vi "Begin.vi"(8 "error in":errorcluster) -> (0 "error out":errorcluster)   [LabVIEW 2014]
doc: "Called before other user functions, this VI is expected to open initial I/O refnums, load in file data, and do all program initialization. Notice that the <B>error out</B> terminal is simply used for data flow. Wiring it to other structures or subVIs ensures that this VI runs first."
uses:
  <vilib>/Rock Robotics/SystemInterfaces/DIO/FPGA_DIOPWMChannel.ctl
  <vilib>/Rock Robotics/WPI/SafetyOutput/WPI_SafetyOutputConfigMenu.ctl
  <vilib>/Rock Robotics/WPI/DriverStation/WPI_DriverStationRobotMode2.ctl
  <vilib>/Rock Robotics/WPI/Joystick/WPI_JoystickDeviceEnum.ctl
  <vilib>/Rock Robotics/WPI/Encoder/WPI_EncoderType.ctl
  <vilib>/Rock Robotics/WPI/RobotDrive/WPI_RobotDriveOpen2MotorWithTalon.vi
  Robot Global Data.vi
  <vilib>/Rock Robotics/Network Tables/SD Write String Array.vi
  <vilib>/Rock Robotics/WPI/MotorControl/WPI_MotorControlOpen Talon.vi
  <vilib>/Rock Robotics/WPI/Solenoid/WPI_SolenoidOpenSingle.vi
  <vilib>/Rock Robotics/WPI/Counter/WPI_CounterDigitalInputToDigitalSource.vi
  LIDAR Present Variable.vi
  <vilib>/express/express arith-compare/Formula/XNode/ExpressFormulaBlockNode.xnode
panel:
  out "Encoder  Ratio 3":dbl
  out "Encoder  Ratio 2":dbl
  out "Encoder  Ratio":dbl
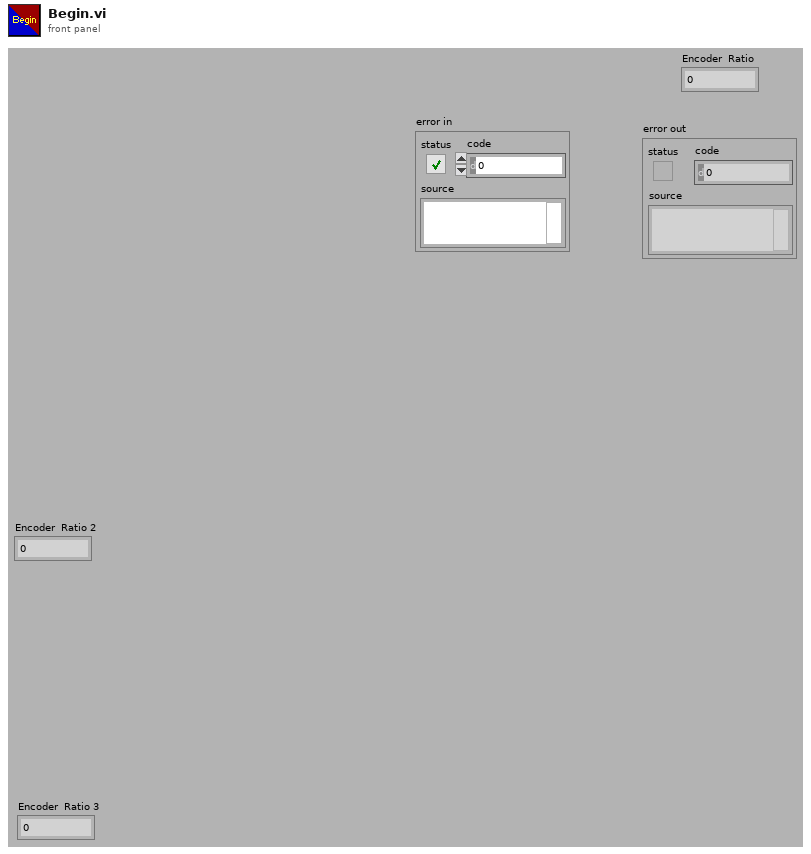
[diagram p1: front panel]
types:
  T1 = enum16{"Solenoid 0", "Solenoid 1", "Solenoid 2", "Solenoid 3", "Solenoid 4"}
  T2 = typedef "WPI_EncoderType.ctl" = enum16{"1x", "2x", "4x"}
  T3 = enum16{"DIO 0", "DIO 1", "DIO 2", "DIO 3", "DIO 4", "DIO 5", "DIO 6", "DIO 7", "DIO 8", "DIO 9"}
  T4 = enum16{"DIO 0", "DIO 1", "DIO 2", "DIO 3", "DIO 4", "DIO 5", "DIO 6", "DIO 7"}
  T5 = enum16{"DIO 0", "DIO 1", "DIO 2", "DIO 3", "DIO 4", "DIO 5", "DIO 6"}
  T6 = typedef "WPI_JoystickDeviceEnum.ctl" = enum16{"USB 0", "USB 1", "USB 2", "USB 3", "USB 4", "USB 5"}
  T7 = enum16{"Solenoid 0", "Solenoid 1", "Solenoid 2", "Solenoid 3", "Solenoid 4", "Solenoid 5"}
  T8 = typedef "FPGA_DIOPWMChannel.ctl" = enum8{"PWM 0", "PWM 1", "PWM 2", "PWM 3", "PWM 4", "PWM 5", "PWM 6", "PWM 7", "PWM 8", "PWM 9", "PWM MXP 0", "PWM MXP 1", "PWM MXP 2", "PWM MXP 3", "PWM MXP 4", "PWM MXP 5", "PWM MXP 6", "PWM MXP 7", "PWM MXP 8", "PWM MXP 9", "Invalid"}
  T9 = typedef "WPI_DriverStationRobotMode2.ctl" = enum16{"Autonomous Disabled", "Autonomous Enabled", "Teleop Disabled", "Teleop Enabled", "Disconnected", "Finish", "Test Disabled", "Test Enabled", "Emergency Stopped"}
  T10 = typedef "WPI_SafetyOutputConfigMenu.ctl" = enum16{"Enable", "Disable"}
  T11 = typedef "WPI_JoystickDevRef.ctl" = cluster{"Device":T6}
  T12 = typedef "WPI_GyroDevRef.ctl" = cluster{"DevStatus":errorcluster, "Analog Module":T13, "Analog Channel":T14, "Offset":dbl, "Gain (VoltsPerDegree/Second)":dbl}
  T13 = typedef "FPGA_TypedefAnalogModule.ctl" = enum16{"Controller 1"}
  T14 = typedef "FPGA_AIChannel.ctl" = enum8{"AI 0", "AI 1", "AI 2", "AI 3", "AI MXP 0", "AI MXP 1", "AI MXP 2", "AI MXP 3", "Invalid"}
  T15 = typedef "WPI_MotorControlDeviceRef.ctl" = cluster{"DeviceStatus":errorcluster, "Type":T16, "PWM":cluster{"Controller":T17, "PWM Channel":T8, "DeadBand":T18}, "CAN":cluster{"Device Number":u8, "Control Mode":T19, "Semaphore":T20, "Max Vout":dbl, "TalonSRX Control Mode":T21}, "Invert":bool, "TransformRef":T22, "InvTransformRef":T22}
  T16 = typedef "WPI_MotorControlType.ctl" = enum16{"PWM", "CAN", "CANTalonSRX"}
  T17 = typedef "FPGA_TypedefDigitalModule.ctl" = enum16{"Controller 1"}
  T18 = typedef "WPI_PWMDeadband.ctl" = cluster{"Name":string, "maxPositivePwm":i32, "minPositivePwm":i32, "centerPwm":i32, "maxNegativePwm":i32, "minNegativePwm":i32, "angularRange":u16}
  T19 = typedef "WPI_CANJaguar_ControlMode.ctl" = enum8{"Percent VBus", "Current", "Speed", "Position", "Voltage"}
  T20 = typedef "Semaphore RefNum" = refnum<k1>
  T21 = typedef "WPI_CANTalonSRX_APIControlMode.ctl" = enum8{"Percent VBus", "Speed", "Position", "Slave", "Unchanged / Invalid"}
  T22 = typedef "WPI_PWMTransform_ConPane.ctl" = refnum<vi>
  T23 = typedef "WPI_RobotDriveDevRef.ctl" = cluster{"DevStatus":errorcluster, "Motors[]":T15[], "Square Inputs":bool, "Max Output":dbl}
  T24 = typedef "WPI_DigitalInputDevRef.ctl" = cluster{"DevStatus":errorcluster, "DIO Channel":T25, "Controller":T17}
  T25 = typedef "FPGA_DIOChannel.ctl" = enum8{"DIO 0", "DIO 1", "DIO 2", "DIO 3", "DIO 4", "DIO 5", "DIO 6", "DIO 7", "DIO 8", "DIO 9", "DIO MXP 0", "DIO MXP 1", "DIO MXP 2", "DIO MXP 3", "DIO MXP 4", "DIO MXP 5", "DIO MXP 6", "DIO MXP 7", "DIO MXP 8", "DIO MXP 9", "DIO MXP 10", "DIO MXP 11", "DIO MXP 12", "DIO MXP 13", "DIO MXP 14", "DIO MXP 15", "Invalid"}
  T26 = typedef "WPI_SolenoidDevRef.ctl" = cluster{"DevStatus":errorcluster, "Pneumatics Control Module":u8, "Forward Solenoid Channel":T27, "Reverse Solenoid Channel":T27}
  T27 = typedef "WPI_SolenoidChannel.ctl" = enum8{"Solenoid 0", "Solenoid 1", "Solenoid 2", "Solenoid 3", "Solenoid 4", "Solenoid 5", "Solenoid 6", "Solenoid 7", "Invalid"}
  T28 = typedef "FPGA_CounterEncoderSourceConvertionLVSourceType.ctl" = cluster{"DevStatus":errorcluster, "AnalogTriggerMode?":bool, "DigitalMode":cluster{"Controller":T17, "DIO Channel":T29}, "AnalogTriggerMode":cluster{"AnalogTriggerIndex":T30, "OutputType":T31}}
  T29 = typedef "FPGA_DIODigitalSourceChannel.ctl" = enum8{"DIO 0", "DIO 1", "DIO 2", "DIO 3", "DIO 4", "DIO 5", "DIO 6", "DIO 7", "DIO 8", "DIO 9", "DIO MXP 0", "DIO MXP 1", "DIO MXP 2", "DIO MXP 3", "DIO MXP 4", "DIO MXP 5", "DIO MXP 6", "DIO MXP 7", "DIO MXP 8", "DIO MXP 9", "DIO MXP 10", "DIO MXP 11", "DIO MXP 12", "DIO MXP 13", "DIO MXP 14", "DIO MXP 15", "Disabled"}
  T30 = typedef "FPGA_AnalogTriggerIndex.ctl" = enum8{"Trig 0", "Trig 1", "Trig 2", "Trig 3", "Trig 4", "Trig 5", "Trig 6", "Trig 7", "Invalid"}
  T31 = typedef "FPGA_AnalogTriggerOutType.ctl" = enum16{"InWindow", "TriggerState", "Rising", "Falling"}
  T32 = typedef "WPI_EncoderDevRef.ctl" = cluster{"DevStatus":errorcluster, "EncoderIndex":T33, "CounterIndex":T34, "DistancePerCount":dbl, "Decoding Type":T2}
  T33 = typedef "FPGA_EncoderIdx.ctl" = enum8{"Enc 0", "Enc 1", "Enc 2", "Enc 3", "Enc 4", "Enc 5", "Enc 6", "Enc 7", "Invalid"}
  T34 = typedef "FPGA_CounterCtrSystemIndex.ctl" = enum8{"Ctr 0", "Ctr 1", "Ctr 2", "Ctr 3", "Ctr 4", "Ctr 5", "Ctr 6", "Ctr 7", "Invalid"}
  T35 = typedef "WPI_I2CDevRef.ctl" = cluster{"DevStatus":errorcluster, "Controller":T17, "Device Address":u8, "Handle":i32, "I2C Bus":T36}
  T36 = typedef "i2c_bus.ctl" = enum16{"I2C On-Board", "I2C MXP", "Invalid"}
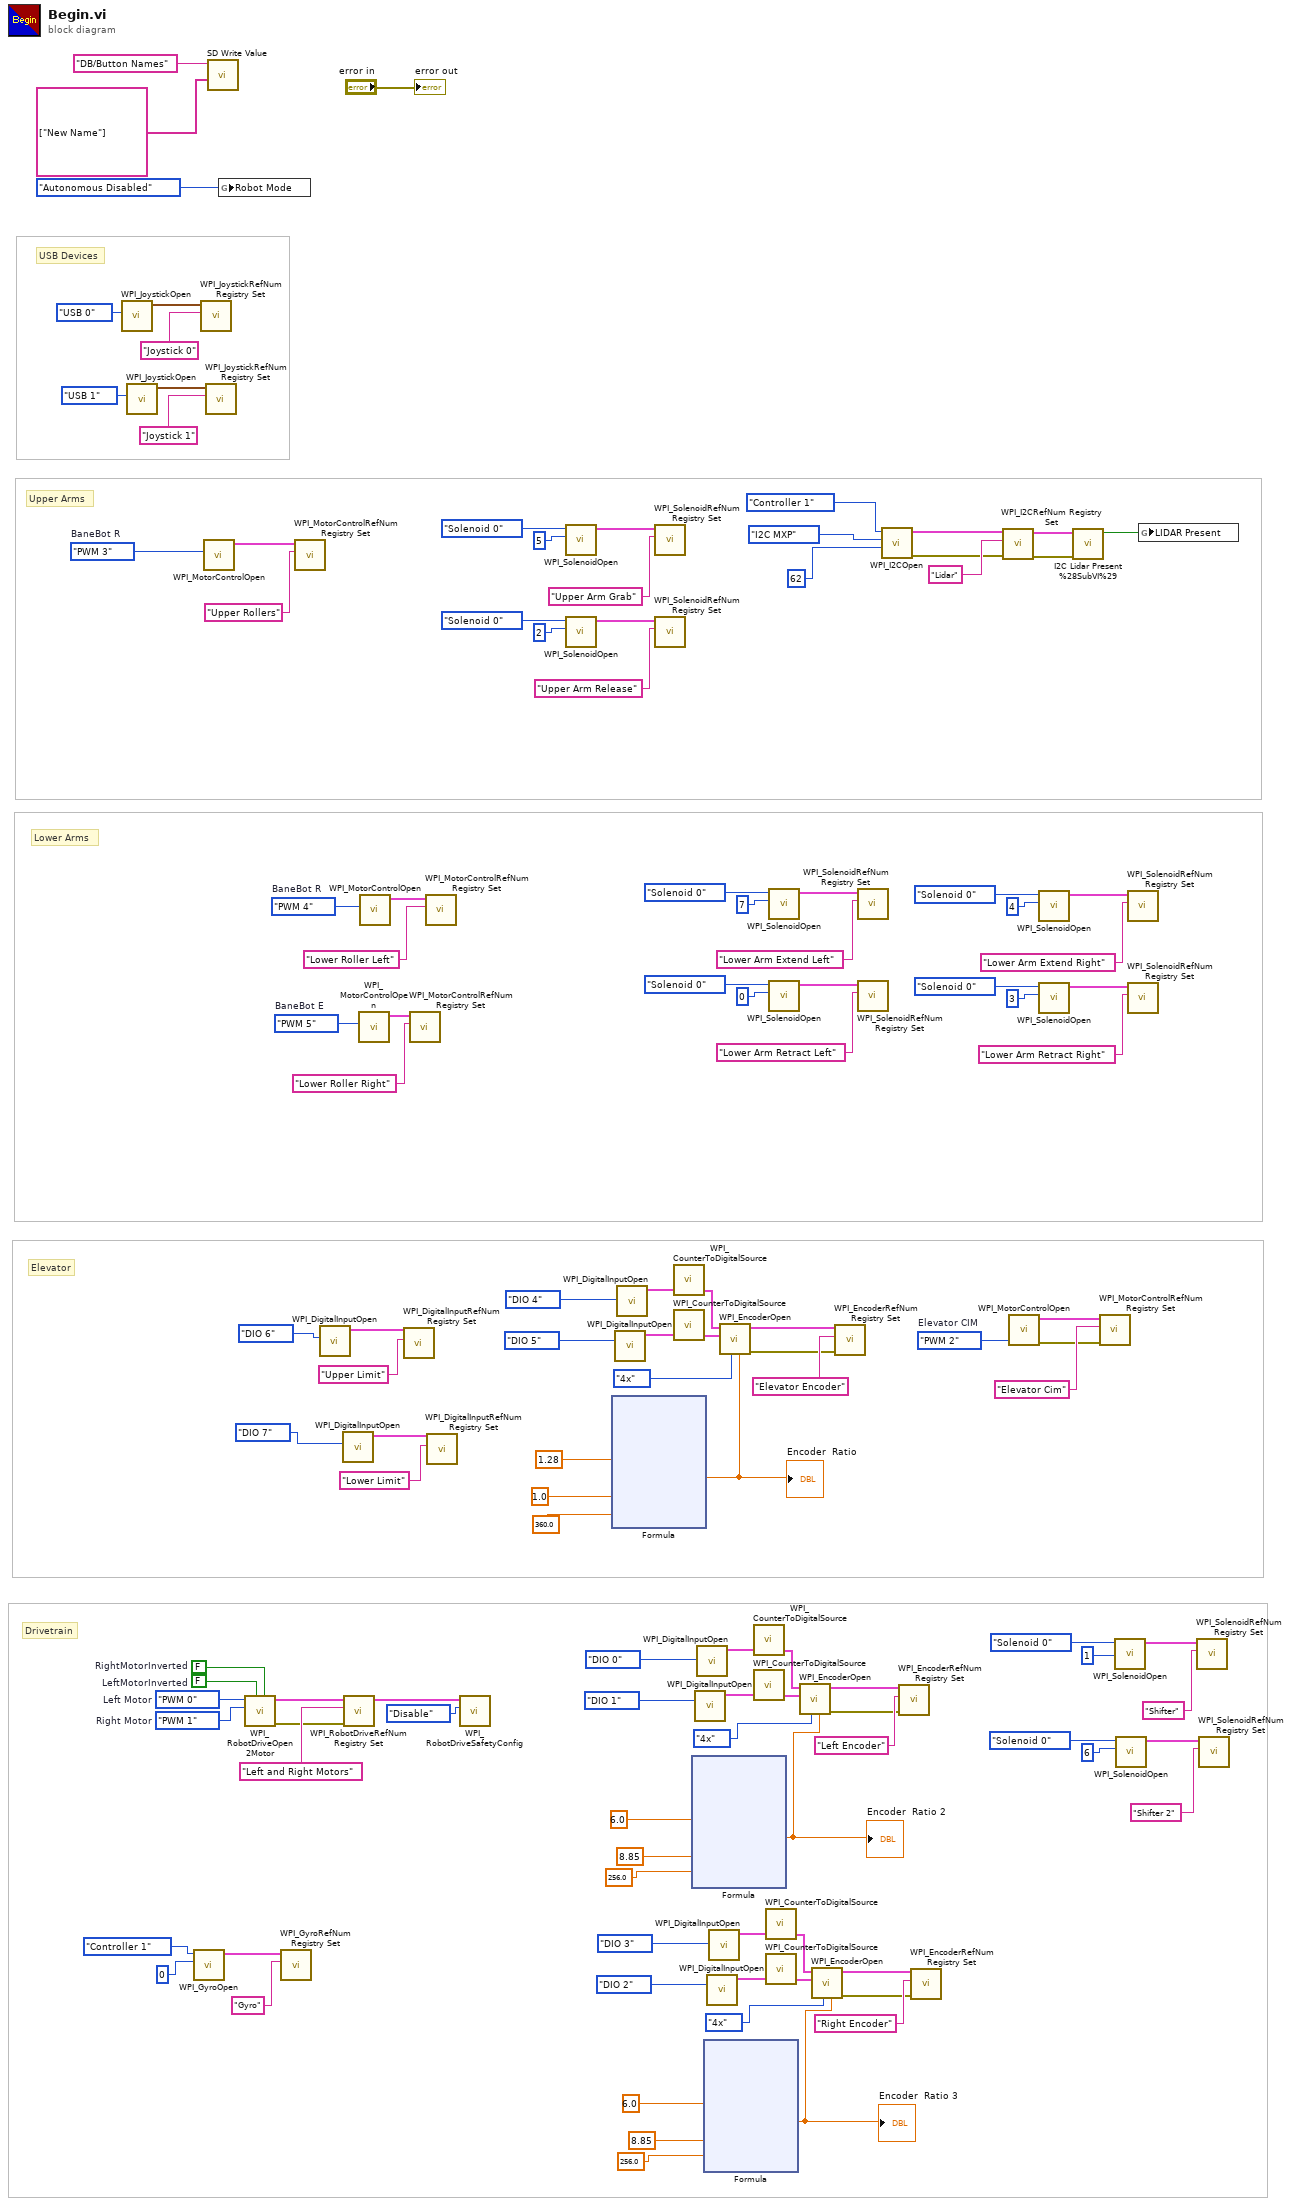
[diagram p0: block diagram]
diagram:
  w98 = FPGA_DIOPWMChannel."PWM 2"  # Elevator CIM
  w102 = FPGA_DIOPWMChannel."PWM 5"  # BaneBot E
  w106 = FPGA_DIOPWMChannel."PWM 4"  # BaneBot R
  w108 = FPGA_DIOPWMChannel."PWM 3"  # BaneBot R
  w119 = FPGA_DIOPWMChannel."PWM 1"  # Right Motor
  w120 = FPGA_DIOPWMChannel."PWM 0"  # Left Motor
  w124 = FALSE  # LeftMotorInverted
  w125 = FALSE  # RightMotorInverted
  # "Upper Arms"
  # "Lower Arms"
  # "Elevator"
  # "Drivetrain"
  # "USB Devices"
  n1 = call <vilib>:"WPI_JoystickOpen.vi"("JoystickDevice"=WPI_JoystickDeviceEnum."USB 0") -> ("JoystickDevRef"=w114:T11)  [unwired: 10 in]
  n2 = call <vilib>:"WPI_JoystickOpen.vi"("JoystickDevice"=WPI_JoystickDeviceEnum."USB 1") -> ("JoystickDevRef"=w79:T11)  [unwired: 10 in]
  n3 = call <vilib>:"WPI_GyroOpen.vi"("Analog Channel"=0, "Controller"=enum16{"Controller 1"}."Controller 1") -> ("GyroDevRef"=w21:T12)  [unwired: 7 in, 2 out]
  n4 = call <vilib>:"WPI_JoystickRefNum Registry Set.vi"("refnum name"="Joystick 0", "JoystickDevRef"=w114) -> ()  [unwired: 8 in, 2 out]
  n5 = call-poly <vilib>:"WPI_MotorControlOpen.vi"("PWM Channel"=w108) -> ("MotorControlDeviceRef"=w109:T15)  [unwired: 9 in, 1 out]
  n6 = call <vilib>:"WPI_JoystickRefNum Registry Set.vi"("refnum name"="Joystick 1", "JoystickDevRef"=w79) -> ()  [unwired: 8 in, 2 out]
  n7 = call-poly <vilib>:"SD Write Value.vi"("String Array"=string[] ["New Name"], "Name"="DB/Button Names") -> ()  [unwired: 8 in, 2 out]
  n8 = global write "Robot Global Data.vi" "Robot Mode"(WPI_DriverStationRobotMode2."Autonomous Disabled" ("Robot Mode")) -> ()
  n9 = call-poly <vilib>:"WPI_RobotDriveOpen2Motor.vi"("Right Motor Inverted"=w125, "Left Motor Inverted"=w124, "Right Motor"=w119, "Left Motor"=w120) -> ("error out"=w121:errorcluster, "RobotDriveDevRef"=w123:T23)  [unwired: 1 in, 5 out]
  n10 = call <vilib>:"WPI_GyroRefNum Registry Set.vi"("refnum name"="Gyro", "GyroDevRef"=w21) -> ()  [unwired: 8 in, 2 out]
  n11 = call <vilib>:"WPI_MotorControlRefNum Registry Set.vi"("refnum name"="Upper Rollers", "MotorControlDevRef"=w109) -> ()  [unwired: 8 in, 2 out]
  n12 = call <vilib>:"WPI_DigitalInputOpen.vi"("DIO Channel"=T5."DIO 6") -> ("DigitalInputDevRef"=w76:T24)  [unwired: 9 in, 1 out]
  n13 = call <vilib>:"WPI_DigitalInputOpen.vi"("DIO Channel"=T4."DIO 7") -> ("DigitalInputDevRef"=w73:T24)  [unwired: 9 in, 1 out]
  n14 = call <vilib>:"WPI_RobotDriveRefNum Registry Set.vi"("error in (no error)"=w121, "refnum name"="Left and Right Motors", "RobotDriveDevRef"=w123) -> ("RobotDriveDevRef"=w118:T23)  [unwired: 8 out]
  n15 = call-poly <vilib>:"WPI_MotorControlOpen.vi"("PWM Channel"=w102) -> ("MotorControlDeviceRef"=w103:T15)  [unwired: 9 in, 1 out]
  n16 = call-poly <vilib>:"WPI_MotorControlOpen.vi"("PWM Channel"=w106) -> ("MotorControlDeviceRef"=w107:T15)  [unwired: 9 in, 1 out]
  n17 = call <vilib>:"WPI_DigitalInputRefNum Registry Set.vi"("refnum name"="Upper Limit", "DigitalInputDevRef"=w76) -> ()  [unwired: 8 in, 2 out]
  n18 = call <vilib>:"WPI_MotorControlRefNum Registry Set.vi"("refnum name"="Lower Roller Right", "MotorControlDevRef"=w103) -> ()  [unwired: 8 in, 2 out]
  n19 = call <vilib>:"WPI_MotorControlRefNum Registry Set.vi"("refnum name"="Lower Roller Left", "MotorControlDevRef"=w107) -> ()  [unwired: 8 in, 2 out]
  n20 = call <vilib>:"WPI_DigitalInputRefNum Registry Set.vi"("refnum name"="Lower Limit", "DigitalInputDevRef"=w73) -> ()  [unwired: 8 in, 2 out]
  n21 = call <vilib>:"WPI_RobotDriveSafetyConfig.vi"("mode"=WPI_SafetyOutputConfigMenu."Disable", "RobotDriveDevRef"=w118) -> ()  [unwired: 8 in, 2 out]
  n22 = call-poly <vilib>:"WPI_SolenoidOpen.vi"("Solenoid Channel"=5, "Pneumatics Control Module (0)"=T1."Solenoid 0") -> ("SolenoidDevRef"=w96:T26)  [unwired: 8 in, 1 out]
  n23 = call-poly <vilib>:"WPI_SolenoidOpen.vi"("Solenoid Channel"=2, "Pneumatics Control Module (0)"=T1."Solenoid 0") -> ("SolenoidDevRef"=w88:T26)  [unwired: 8 in, 1 out]
  n24 = xnode "Formula"("Wheel Diameter"=1.28, "Gear Ratio"=1.0, "PPR"=360.0) -> ("Result"=w58:dbl)  [unwired: 1 in, 1 out]
  "Encoder  Ratio" <- w58
  n25 = call <vilib>:"WPI_DigitalInputOpen.vi"("DIO Channel"=T3."DIO 5") -> ("DigitalInputDevRef"=w62:T24)  [unwired: 9 in, 1 out]
  n26 = call <vilib>:"WPI_DigitalInputOpen.vi"("DIO Channel"=T3."DIO 4") -> ("DigitalInputDevRef"=w63:T24)  [unwired: 9 in, 1 out]
  n27 = call <vilib>:"WPI_SolenoidRefNum Registry Set.vi"("refnum name"="Upper Arm Grab", "SolenoidDevRef"=w96) -> ()  [unwired: 8 in, 2 out]
  n28 = call <vilib>:"WPI_SolenoidRefNum Registry Set.vi"("refnum name"="Upper Arm Release", "SolenoidDevRef"=w88) -> ()  [unwired: 8 in, 2 out]
  n29 = call-poly <vilib>:"WPI_CounterToDigitalSource.vi"("DigitalInputDevRef"=w63) -> ("Digital Source"=w70:T28)  [unwired: 6 out]
  n30 = call-poly <vilib>:"WPI_CounterToDigitalSource.vi"("DigitalInputDevRef"=w62) -> ("Digital Source"=w71:T28)  [unwired: 6 out]
  n31 = xnode "Formula"("Wheel Diameter"=6.0, "Gear Ratio"=8.85, "PPR"=256.0) -> ("Result"=w44:dbl)  [unwired: 1 in, 1 out]
  "Encoder  Ratio 2" <- w44
  n32 = call <vilib>:"WPI_DigitalInputOpen.vi"("DIO Channel"=T3."DIO 1") -> ("DigitalInputDevRef"=w48:T24)  [unwired: 9 in, 1 out]
  n33 = call <vilib>:"WPI_DigitalInputOpen.vi"("DIO Channel"=T3."DIO 0") -> ("DigitalInputDevRef"=w49:T24)  [unwired: 9 in, 1 out]
  n34 = xnode "Formula"("Wheel Diameter"=6.0, "Gear Ratio"=8.85, "PPR"=256.0) -> ("Result"=w30:dbl)  [unwired: 1 in, 1 out]
  "Encoder  Ratio 3" <- w30
  n35 = call <vilib>:"WPI_DigitalInputOpen.vi"("DIO Channel"=T3."DIO 2") -> ("DigitalInputDevRef"=w34:T24)  [unwired: 9 in, 1 out]
  n36 = call <vilib>:"WPI_DigitalInputOpen.vi"("DIO Channel"=T3."DIO 3") -> ("DigitalInputDevRef"=w35:T24)  [unwired: 9 in, 1 out]
  n37 = call <vilib>:"WPI_EncoderOpen.vi"("DistancePerCount"=w58, "Decoding Type"=WPI_EncoderType."4x", "BSource"=w71, "ASource"=w70) -> ("error out"=w60:errorcluster, "EncoderDevRef"=w61:T32)  [unwired: 4 in, 2 out]
  n38 = call-poly <vilib>:"WPI_CounterToDigitalSource.vi"("DigitalInputDevRef"=w49) -> ("Digital Source"=w56:T28)  [unwired: 6 out]
  n39 = call-poly <vilib>:"WPI_CounterToDigitalSource.vi"("DigitalInputDevRef"=w48) -> ("Digital Source"=w57:T28)  [unwired: 6 out]
  n40 = call-poly <vilib>:"WPI_CounterToDigitalSource.vi"("DigitalInputDevRef"=w35) -> ("Digital Source"=w42:T28)  [unwired: 6 out]
  n41 = call-poly <vilib>:"WPI_CounterToDigitalSource.vi"("DigitalInputDevRef"=w34) -> ("Digital Source"=w43:T28)  [unwired: 6 out]
  n42 = call-poly <vilib>:"WPI_SolenoidOpen.vi"("Solenoid Channel"=7, "Pneumatics Control Module (0)"=T1."Solenoid 0") -> ("SolenoidDevRef"=w28:T26)  [unwired: 8 in, 1 out]
  n43 = call-poly <vilib>:"WPI_SolenoidOpen.vi"("Solenoid Channel"=0, "Pneumatics Control Module (0)"=T1."Solenoid 0") -> ("SolenoidDevRef"=w25:T26)  [unwired: 8 in, 1 out]
  n44 = call <vilib>:"WPI_EncoderOpen.vi"("DistancePerCount"=w44, "Decoding Type"=WPI_EncoderType."4x", "BSource"=w57, "ASource"=w56) -> ("error out"=w46:errorcluster, "EncoderDevRef"=w47:T32)  [unwired: 4 in, 2 out]
  n45 = call <vilib>:"WPI_EncoderOpen.vi"("DistancePerCount"=w30, "Decoding Type"=WPI_EncoderType."4x", "BSource"=w43, "ASource"=w42) -> ("error out"=w32:errorcluster, "EncoderDevRef"=w33:T32)  [unwired: 4 in, 2 out]
  n46 = call <vilib>:"WPI_EncoderRefNum Registry Set.vi"("error in (no error)"=w60, "refnum name"="Elevator Encoder", "EncoderDevRef"=w61) -> ()  [unwired: 7 in, 2 out]
  n47 = call <vilib>:"WPI_SolenoidRefNum Registry Set.vi"("refnum name"="Lower Arm Extend Left", "SolenoidDevRef"=w28) -> ()  [unwired: 8 in, 2 out]
  n48 = call <vilib>:"WPI_SolenoidRefNum Registry Set.vi"("refnum name"="Lower Arm Retract Left", "SolenoidDevRef"=w25) -> ()  [unwired: 8 in, 2 out]
  n49 = call <vilib>:"WPI_I2COpen.vi"("Device Address"=62, "I2C Bus"=enum16{"I2C On-Board", "I2C MXP"}."I2C MXP", "Controller"=enum16{"Controller 1", "Controller 2"}."Controller 1") -> ("error out"=w13:errorcluster, "I2CDevRef"=w18:T35)  [unwired: 7 in]
  n50 = call <vilib>:"WPI_EncoderRefNum Registry Set.vi"("error in (no error)"=w46, "refnum name"="Left Encoder", "EncoderDevRef"=w47) -> ()  [unwired: 7 in, 2 out]
  n51 = call <vilib>:"WPI_EncoderRefNum Registry Set.vi"("error in (no error)"=w32, "refnum name"="Right Encoder", "EncoderDevRef"=w33) -> ()  [unwired: 7 in, 2 out]
  n52 = call <vilib>:"WPI_I2CRefNum Registry Set.vi"("error in (no error)"=w13, "refnum name"="Lidar", "I2CDevRef"=w18) -> ("error out"=w11:errorcluster, "I2CDevRef"=w12:T35)  [unwired: 7 in]
  n53 = call-poly <vilib>:"WPI_MotorControlOpen.vi"("PWM Channel"=w98) -> ("error out"=w99:errorcluster, "MotorControlDeviceRef"=w93:T15)  [unwired: 9 in]
  n54 = call-poly <vilib>:"WPI_SolenoidOpen.vi"("Solenoid Channel"=4, "Pneumatics Control Module (0)"=T1."Solenoid 0") -> ("SolenoidDevRef"=w8:T26)  [unwired: 8 in, 1 out]
  n55 = call-poly <vilib>:"WPI_SolenoidOpen.vi"("Solenoid Channel"=3, "Pneumatics Control Module (0)"=T1."Solenoid 0") -> ("SolenoidDevRef"=w5:T26)  [unwired: 8 in, 1 out]
  n56 = call "I2C Lidar Present %28SubVI%29.vi"("error in (no error)"=w11, "I2CDevRef"=w12) -> ("Sensor Present"=w10:bool)  [unwired: 9 in]
  n57 = call <vilib>:"WPI_MotorControlRefNum Registry Set.vi"("error in (no error)"=w99, "refnum name"="Elevator Cim", "MotorControlDevRef"=w93) -> ()  [unwired: 7 in, 2 out]
  n58 = call-poly <vilib>:"WPI_SolenoidOpen.vi"("Solenoid Channel"=1, "Pneumatics Control Module (0)"=T1."Solenoid 0") -> ("SolenoidDevRef"=w91:T26)  [unwired: 8 in, 1 out]
  n59 = call-poly <vilib>:"WPI_SolenoidOpen.vi"("Solenoid Channel"=6, "Pneumatics Control Module (0)"=T7."Solenoid 0") -> ("SolenoidDevRef"=w84:T26)  [unwired: 8 in, 1 out]
  n60 = call <vilib>:"WPI_SolenoidRefNum Registry Set.vi"("refnum name"="Lower Arm Extend Right", "SolenoidDevRef"=w8) -> ()  [unwired: 8 in, 2 out]
  n61 = call <vilib>:"WPI_SolenoidRefNum Registry Set.vi"("refnum name"="Lower Arm Retract Right", "SolenoidDevRef"=w5) -> ()  [unwired: 8 in, 2 out]
  n62 = global write "LIDAR Present Variable.vi" "LIDAR Present"(w10) -> ()
  n63 = call <vilib>:"WPI_SolenoidRefNum Registry Set.vi"("refnum name"="Shifter", "SolenoidDevRef"=w91) -> ()  [unwired: 8 in, 2 out]
  n64 = call <vilib>:"WPI_SolenoidRefNum Registry Set.vi"("refnum name"="Shifter 2", "SolenoidDevRef"=w84) -> ()  [unwired: 8 in, 2 out]
  "error out" <- "error in"
